vi "Items to MCLB Item Names.vi"(7 "Items":T1[](array[typedef])) -> (3 "Item Names":string[][](array[string]))   [LabVIEW 2019, in "Selector.lvclass"]
uses:
  Selector.lvclass
  Item.ctl
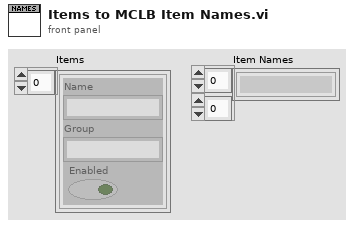
[diagram p1: front panel]
types:
  T1 = typedef "Selector.lvclass/Item.ctl" = cluster{"Name":string, "Group":string, "Enabled":bool}
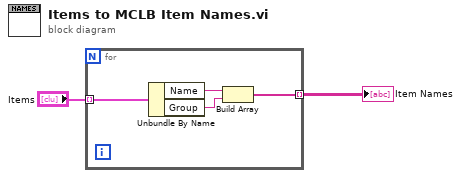
[diagram p0: block diagram]
diagram:
  n1 = for {
    tunnel: "Items" -> [w6] mode=indexing
    tunnel: [w3] -> w1 mode=indexing
    n2 = Unbundle By Name(w6) -> ("Name"=w5:string, "Group"=w4:string)
    n3 = Build Array(w5, w4) -> (w3:string[])
  }
  "Item Names" <- w1
